vi "Estrazione fondo - Host.vi"(4 "polynomial order":i32=3, 5 "LowPass Filter: Low cutoff frequency":dbl=20000.0 format="%#_13g", 6 "side points":i32=6, 7 "PolyFitting: Poly Grade":dbl=5.0, 8 "Low Pass filter: Sampling freq: fs":dbl=30000000.0 format="%#_13g", 9 "SubtractionType":T1(ring), 10 "error in":errorcluster, 11 "FPGA VI Reference In":refnum<k20>) -> (0 "Residual Signal":dbl[](graph), 1 "Complete Mean Signal":dbl[](graph), 2 "error out":errorcluster, 3 "FPGA VI Reference Out":refnum<k20>)   [LabVIEW 2014]
uses:
  <vilib>/Analysis/3filter.llb/Filter Passband Type.ctl
  <vilib>/Analysis/3filter.llb/Savitzky-Golay Filter (DBL).vi
  <vilib>/Utility/error.llb/Error Cluster From Error Code.vi
  <vilib>/RVI Host/nirviSupport.llb/nirviErrorClusterFromErrorCode.vi
  <vilib>/rvi/errors/niLvFpgaAdjustHostInterfaceError.vi
  <vilib>/Analysis/3filter.llb/Butterworth Filter (DBL).vi
  <vilib>/rvi/interface/nirviMethod/nirviMethod.xnode
  <vilib>/rvi/errors/niLvFpgaMergeErrorWithErrorCode.vi
  <vilib>/FPGAPlugInAG/Dynamic/niLvFpga_AcknowledgeIrq_Dynamic.vi
  <vilib>/rvi/interface/nirviMethod/StockFPGA_InlinedMethodWaitForSingleIRQ.vi
  <vilib>/FPGAPlugInAG/Dynamic/niLvFpga_WaitOnIrq_Dynamic.vi
  <vilib>/Analysis/NI_AALBase.lvlib
  <vilib>/FPGAPlugInAG/Dynamic/niLvFpga_ReadFifo_Dynamic.vi
  <vilib>/FPGAPlugInAG/Dynamic/niLvFpga_WriteFifo_Dynamic.vi
panel:
  # "SavGolay"
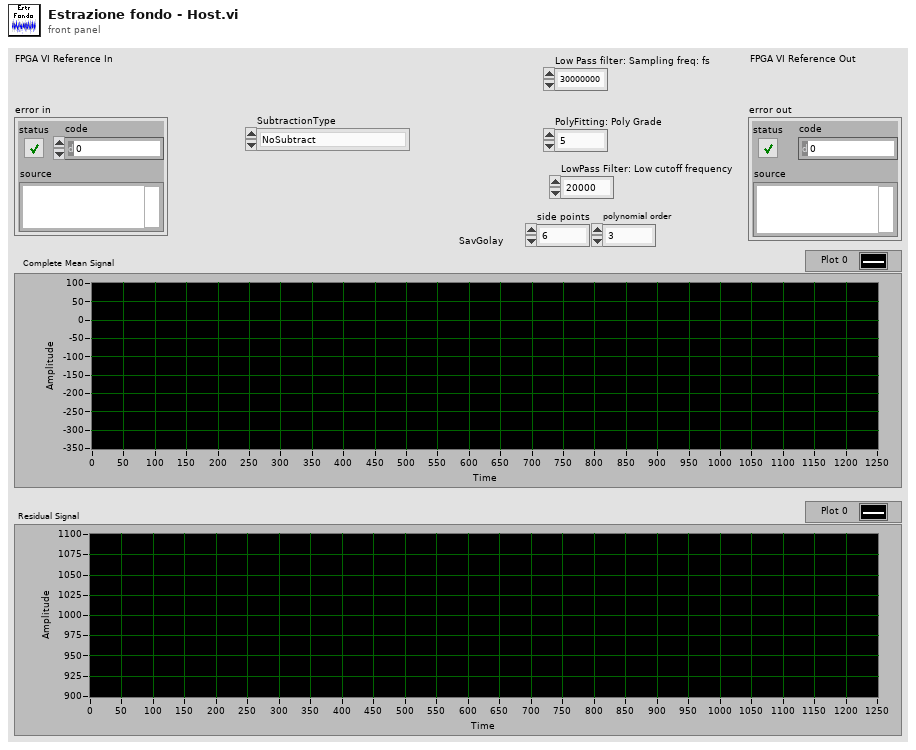
[diagram p1: front panel]
types:
  T1 = enum16{"NoSubtract", "StartingCurve", "LowPass", "PolyFitting", "SavGolay"}
  T2 = typedef "NI_AALBase.lvlib/Filter Passband Type.ctl" = enum32{"Lowpass", "Highpass", "Bandpass", "Bandstop"}
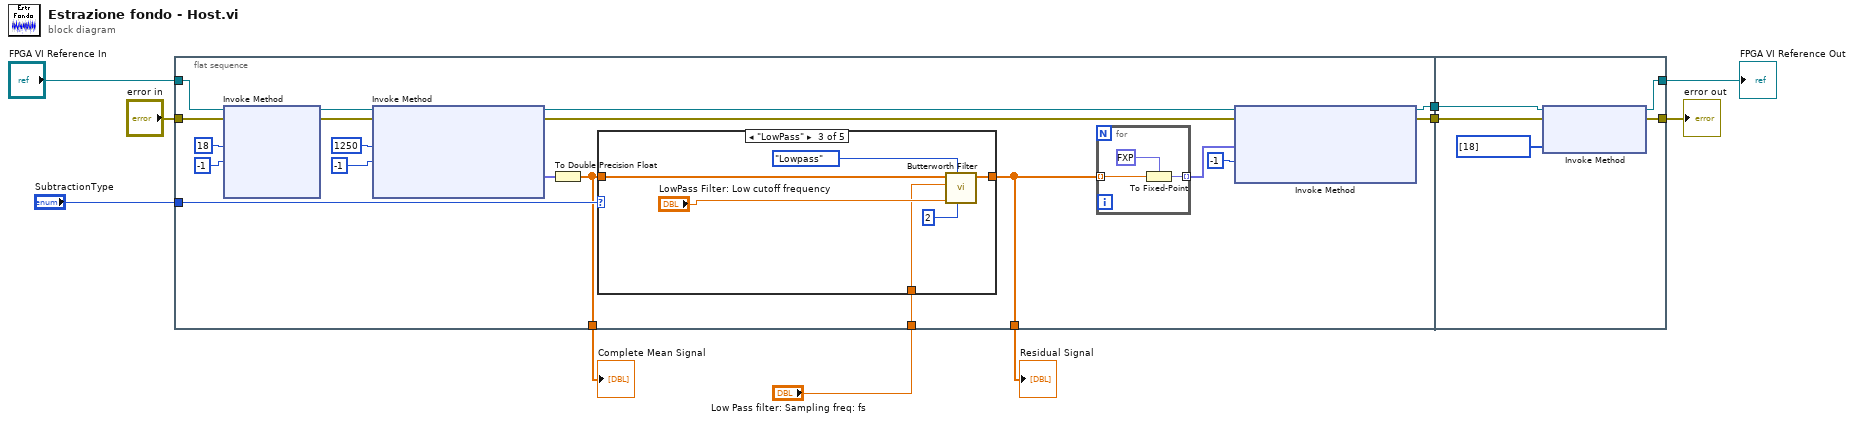
[diagram p0: block diagram]
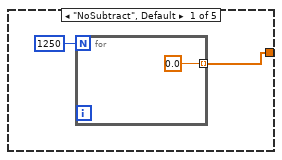
[diagram p2: hidden frame]
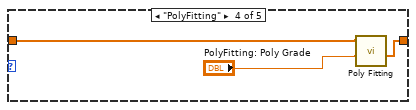
[diagram p4: hidden frame]
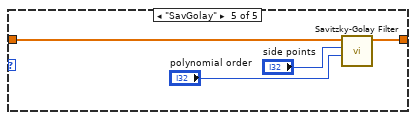
[diagram p5: hidden frame]
diagram:
  n1 = flat-sequence {
    tunnel: [w24] -> w10
    tunnel: [w23] -> w9
    tunnel: "error in" -> [w16]
    tunnel: "FPGA VI Reference In" -> [w15]
    tunnel: "SubtractionType" -> [w14]
    tunnel: [w13] -> w3
    tunnel: [w12] -> w2
    tunnel: "Low Pass filter: Sampling freq: fs" -> [w11]
    tunnel: w10 -> [w54]
    tunnel: w9 -> [w53]
    tunnel: [w51] -> w5
    tunnel: [w50] -> w6
    frame #0 {
      n2 = xnode "Invoke Method"("FPGA VI Reference In"=w15, "error in"=w16, "IRQ Number(s)"=18, "Timeout (ms)"=-1) -> ("FPGA VI Reference Out"=w19:refnum<k20>, "error out"=w18:errorcluster)  [unwired: 2 out]
      n3 = xnode "Invoke Method"("FPGA VI Reference In"=w19, "error in"=w18, "Number of Elements"=u32 1250, "Timeout (ms)"=-1) -> ("FPGA VI Reference Out"=w27:refnum<k20>, "error out"=w26:errorcluster, "Data"=w20:fxp<+,44,44>[])  [unwired: 1 out]
      n4 = To Double Precision Float(number=w20) -> (double precision float=w13:dbl[])
      n5 = case shown="\"LowPass\"" w14 {
        tunnel: [w30 w33 w35 w40 w45] -> w12
        tunnel: w13 -> [_ w33 w36 w42 w46]
        tunnel: w11 -> [_ _ w34 _ _]
        frame "NoSubtract", Default {
          n6 = for {
            N: 1250 -> [_]
            tunnel: [0.0 ("sampling freq: fs")] -> w30 mode=indexing
          }
        }
        frame "StartingCurve" {
        }
        frame "LowPass" {
          n7 = call-poly <vilib>:"Butterworth Filter.vi"("order"=2, "filter type"=Filter_Passband_Type."Lowpass", "low cutoff freq: fl"="LowPass Filter: Low cutoff frequency", "sampling freq: fs"=w34, "X"=w36) -> ("Filtered X"=w35:dbl[])  [unwired: 3 in, 1 out]
        }
        frame "PolyFitting" {
          n8 = call "Poly Fitting.vi"("Poly Grade"="PolyFitting: Poly Grade", "Signal"=w42) -> ("Poly Signal"=w40:dbl[])  [unwired: 8 in, 1 out]
        }
        frame "SavGolay" {
          n9 = call-poly <vilib>:"Savitzky-Golay Filter.vi"("polynomial order"="polynomial order", "side points"="side points", "X"=w46) -> ("Filtered X"=w45:dbl[])  [unwired: 7 in, 1 out]
        }
      }
      n10 = for {
        tunnel: w12 -> [w49] mode=indexing
        tunnel: [w47] -> w25 mode=indexing
        n11 = To Fixed-Point(fixed-point type=fxp<+/-,12,12> 0.0, number=w49) -> (fixed-point=w47:fxp<+/-,12,12>)
      }
      n12 = xnode "Invoke Method"("FPGA VI Reference In"=w27, "error in"=w26, "Data"=w25, "Timeout (ms)"=-1) -> ("FPGA VI Reference Out"=w24:refnum<k20>, "error out"=w23:errorcluster)  [unwired: 1 out]
    }
    frame #1 {
      n13 = xnode "Invoke Method"("FPGA VI Reference In"=w54, "error in"=w53, "IRQ Number(s)"=i32[] [18]) -> ("FPGA VI Reference Out"=w50:refnum<k20>, "error out"=w51:errorcluster)
    }
  }
  "FPGA VI Reference Out" <- w6
  "error out" <- w5
  "Residual Signal" <- w2
  "Complete Mean Signal" <- w3
